vi "Bracket Balancing.VI"(1 "string before":string) -> (0 "string after":string)   [LabVIEW 2020, in "NI_Gmath.lvlib"]
uses:
  NI_Gmath.lvlib
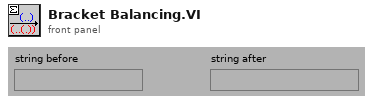
[diagram p1: front panel]
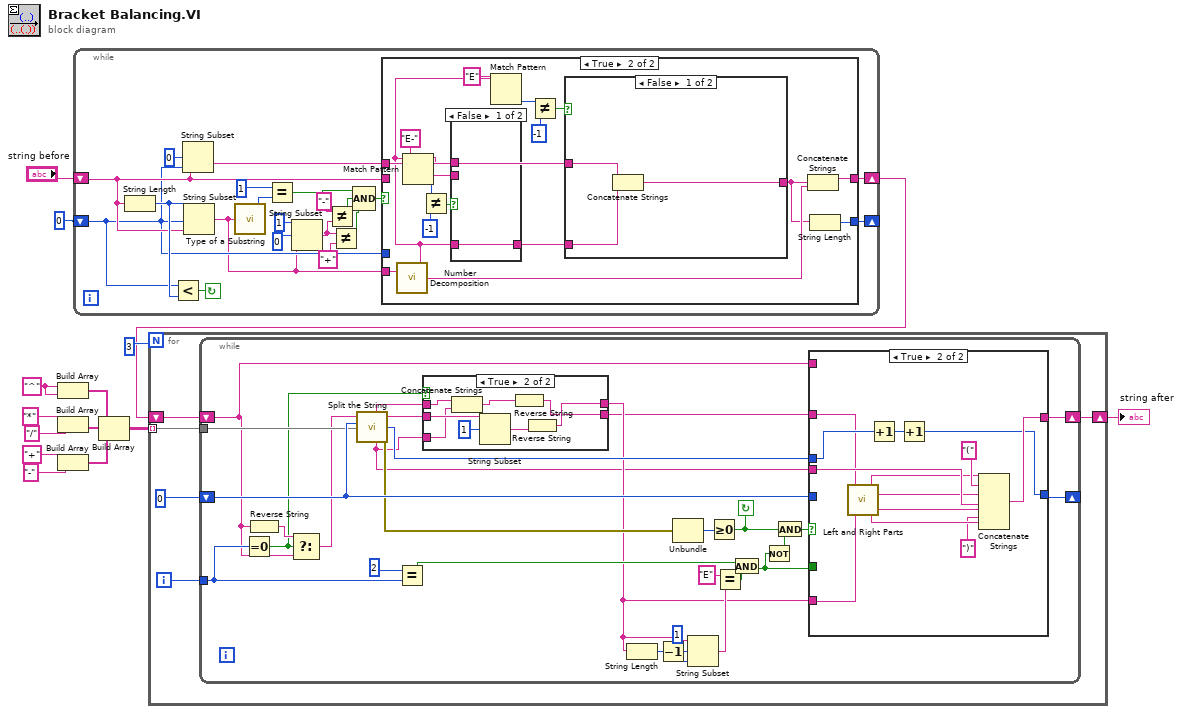
[diagram p0: block diagram]
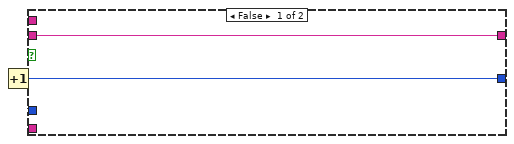
[diagram p2: hidden frame]
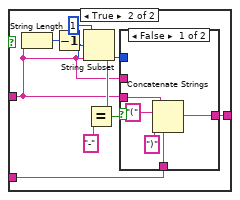
[diagram p3: hidden frame]
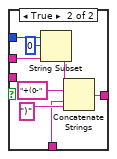
[diagram p4: hidden frame]
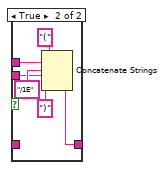
[diagram p5: hidden frame]
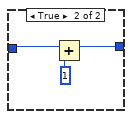
[diagram p8: hidden frame]
diagram:
  w5 = "^"
  n1 = Build Array(w5, w5) -> (w9:string[])
  n2 = Build Array("*", "/") -> (w8:string[])
  n3 = Build Array("+", "-") -> (w7:string[])
  n4 = while {
    shift-left: "string before" -> [w28]
    shift-right: [w25] -> w1
    shift-left: 0 -> [w26]
    shift-right: [w31] -> _
    stop <- w29 continue-if-true
    n5 = String Length(string=w28) -> (length=w30:i32)
    n6 = Less?(x=w26, y=w30) -> (x < y?=w29:bool)
    n7 = String Subset(string=w28, offset (0)=0, length (rest)=w26) -> (substring=w27:string)
    n8 = String Subset(string=w28, offset (0)=w26, length (rest)=w30) -> (substring=w24:string)
    n9 = call "Type of a Substring.VI"("item"=w24) -> ("type"=w32:i32)
    n10 = Equal?(x=1, y=w32) -> (x = y?=w20:bool)
    n11 = String Subset(string=w24, offset (0)=0, length (rest)=1) -> (substring=w19:string)
    n12 = Not Equal?(x="-", y=w19) -> (x != y?=w17:bool)
    n13 = Not Equal?(x=w19, y="+") -> (x != y?=w18:bool)
    n14 = Compound Arithmetic op=AND(w20, w17, w18) -> (w21:bool)
    n15 = case shown="True" w21 {
      tunnel: w26 -> [w37 _]
      tunnel: [w36 w51] -> w31
      tunnel: w28 -> [w35 _]
      tunnel: [w35 w53] -> w25
      tunnel: w24 -> [_ w55]
      tunnel: w27 -> [_ w50]
      frame False {
        n16 = Increment(x=w37) -> (x+1=w36:i32)
      }
      frame True {
        n17 = call "Number Decomposition.VI"("number string"=w55) -> ("number"=w42:string, "rest"=w54:string)  [unwired: 1 in, 1 out]
        n18 = Match Pattern(string=w42, regular expression="E-") -> (before substring=w48:string, after substring=w49:string, offset past match=w45:i32)  [unwired: 1 in, 1 out]
        n19 = Not Equal?(x=w45, y=-1) -> (x != y?=w47:bool)
        n20 = case shown="False" w47 {
          tunnel: w42 -> [w81 _]
          tunnel: [w81 w83] -> w43
          tunnel: w48 -> [_ w86]
          tunnel: w49 -> [_ w84]
          frame False {
          }
          frame True {
            n21 = Concatenate Strings("(", w86, "/1E", w84, ")") -> (w83:string)
          }
        }
        n22 = Match Pattern(string=w42, regular expression="E") -> (offset past match=w40:i32)  [unwired: 1 in, 3 out]
        n23 = Not Equal?(x=w40, y=-1) -> (x != y?=w39:bool)
        n24 = case shown="False" w39 {
          tunnel: w43 -> [w56 w67]
          tunnel: w50 -> [w58 w60]
          tunnel: [w57 w62] -> w52
          frame False {
            n25 = Concatenate Strings(w58, w56) -> (w57:string)
          }
          frame True {
            n26 = String Length(string=w60) -> (length=w66:i32)
            n27 = Decrement(x=w66) -> (x-1=w59:i32)
            n28 = String Subset(string=w60, offset (0)=w59, length (rest)=1) -> (substring=w61:string)
            n29 = Equal?(x=w61, y="-") -> (x = y?=w63:bool)
            n30 = case shown="False" w63 {
              tunnel: w60 -> [w72 _]
              tunnel: [w71 w80] -> w62
              tunnel: w67 -> [w68 w77]
              tunnel: w60 -> [_ w76]
              tunnel: w59 -> [_ w74]
              frame False {
                n31 = Concatenate Strings(w72, "(", w68, ")") -> (w71:string)
              }
              frame True {
                n32 = String Subset(string=w76, offset (0)=0, length (rest)=w74) -> (substring=w73:string)
                n33 = Concatenate Strings(w73, "+(0-", w77, ")") -> (w80:string)
              }
            }
          }
        }
        n34 = Concatenate Strings(w52, w54) -> (w53:string)
        n35 = String Length(string=w52) -> (length=w51:i32)
      }
    }
  }
  n36 = Build Array(w9, w8, w7) -> (w13:string[][])
  n37 = for {
    N: 3 -> [_]
    shift-right: [w88] -> w2
    shift-left: w1 -> [w91]
    tunnel: w13 -> [w92] mode=indexing
    i -> [w89]
    n38 = while {
      tunnel: w89 -> [w102]
      tunnel: w92 -> [w109]
      shift-left: 0 -> [w112]
      shift-right: [w121] -> _
      shift-left: w91 -> [w100]
      shift-right: [w105] -> w88
      stop <- w106 continue-if-true
      n39 = Equal To 0?(x=w102) -> (x = 0?=w93:bool)
      n40 = Reverse String(1:w100) -> (0:w101:string)
      n41 = Select(t=w101, s=w93, f=w100) -> (s? t:f=w99:string)
      n42 = call "Split the String.vi"("Marker"=w109, "position"=w112, "string"=w99) -> ("error out"=w111:errorcluster, "choice"=w94:string, "new position"=w113:i32, "after"=w96:string, "before"=w98:string)  [unwired: 1 in]
      n43 = Equal?(x=2, y=w102) -> (x = y?=w115:bool)
      n44 = case shown="True" w93 {
        tunnel: w98 -> [w123 w128]
        tunnel: [w123 w129] -> w97
        tunnel: w96 -> [w122 w131]
        tunnel: [w122 w125] -> w95
        tunnel: w94 -> [_ w127]
        frame False {
        }
        frame True {
          n45 = Concatenate Strings(w128, w127) -> (w126:string)
          n46 = String Subset(string=w131, offset (0)=1) -> (substring=w130:string)  [unwired: 1 in]
          n47 = Reverse String(1:w126) -> (0:w125:string)
          n48 = Reverse String(1:w130) -> (0:w129:string)
        }
      }
      n49 = String Length(string=w97) -> (length=w119:i32)
      n50 = Decrement(x=w119) -> (x-1=w118:i32)
      n51 = Unbundle(w111) -> ("code"=w110:i32)  [unwired: 2 out]
      n52 = String Subset(string=w97, offset (0)=w118, length (rest)=1) -> (substring=w104:string)
      n53 = Greater Or Equal To 0?(x=w110) -> (x >= 0?=w106:bool)
      n54 = Equal?(x="E", y=w104) -> (x = y?=w116:bool)
      n55 = And(x=w115, y=w116) -> (x .and. y?=w107:bool)
      n56 = Not(x=w107) -> (.not. x?=w114:bool)
      n57 = And(x=w106, y=w114) -> (x .and. y?=w108:bool)
      n58 = case shown="True" w108 {
        tunnel: w95 -> [_ w145]
        tunnel: w97 -> [_ w141]
        tunnel: [w135 w142] -> w105
        tunnel: w94 -> [_ w151]
        tunnel: [w132 w140] -> w121
        tunnel: w112 -> [w133 _]
        tunnel: w100 -> [w135 _]
        tunnel: w113 -> [_ w146]
        tunnel: w107 -> [w134 _]
        frame False {
          n59 = case shown="False" w134 {
            tunnel: w133 -> [w136 w139]
            tunnel: [w136 w137] -> w132
            frame False {
            }
            frame True {
              n60 = Add(x=w139, y=1) -> (x+y=w137:i32)
            }
          }
        }
        frame True {
          n61 = call "Left and Right Parts.vi"("after"=w145, "before"=w141) -> ("left start"=w143:string, "left end"=w144:string, "right start"=w148:string, "right end"=w150:string)
          n62 = Increment(x=w146) -> (x+1=w152:i32)
          n63 = Increment(x=w152) -> (x+1=w140:i32)
          n64 = Concatenate Strings(w143, "(", w144, w151, w148, ")", w150) -> (w142:string)
        }
      }
    }
  }
  "string after" <- w2
